vi "__fetchcount.vi"(10 "Numeric":i32, 11 "Numeric 2":u32) -> (3 "Boolean":bool)   [LabVIEW 2017]
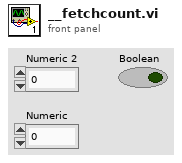
[diagram p1: front panel]
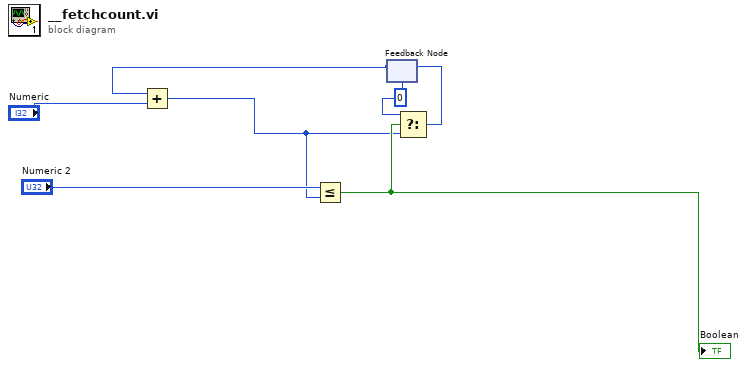
[diagram p0: block diagram]
diagram:
  w1 = u32 0
  n1 = feedback #1(w1) -> (w3:u32)
  n2 = Add(x=w3, y="Numeric") -> (x+y=w4:u32)
  n3 = Less Or Equal?(x="Numeric 2", y=w4) -> (x <= y?=w6:bool)
  "Boolean" <- w6
  n4 = Select(t=w1, s=w6, f=w4) -> (s? t:f=w2:u32)
  n5 = feedback-in #1(w2) -> ()
